vi "Create All Message Queues.vi"(8 "error in (no error)":errorcluster caption="에러 입력(에러 없음)") -> (0 "error out":errorcluster caption="에러 출력", 3 "Message Queues out":T1 caption="메시지 큐 출력")   [LabVIEW 2018, in "Message Queue.lvlib"]
doc: "이 VI는 어플리케이션의 모든 메시지 큐를 생성하고 초기화합니다. 어플리케이션에 하나 이상의 메시지 큐가 필요하면, 위의 \"메시지 큐\" 상수에서 마우스 오른쪽 버튼을 클릭한 후 타입 정의 열기를 선택합니다. 타입 정의에 새 메시지 큐를 추가한 후, 이 VI에서 초기화합니다."
uses:
  Message Queue.lvlib
  All Message Queues.ctl
  Message Cluster.ctl
  Enqueue Message (Single).vi
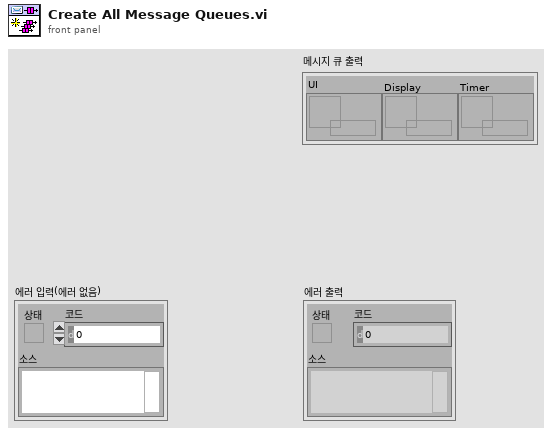
[diagram p1: front panel]
types:
  T1 = typedef "Message Queue.lvlib/All Message Queues.ctl" = cluster{"UI":refnum<queue>, "Display":refnum<queue>, "Timer":refnum<queue>}
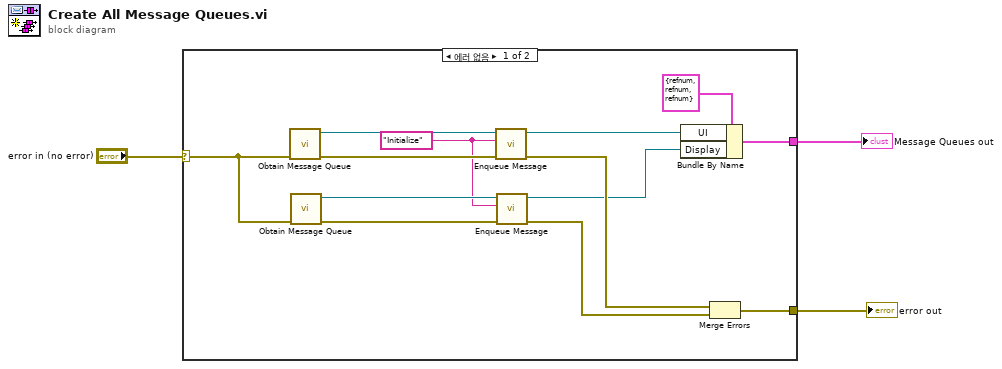
[diagram p0: block diagram]
diagram:
  n1 = case shown="에러 없음" "error in (no error)" {
    selector: "error in (no error)" -> [w5 w17]
    tunnel: [w9 w17] -> w3
    tunnel: [w6 _] -> w2
    frame No Error {
      w4 = "Initialize" ("Message")
      n2 = call "Obtain Message Queue.vi"("error in (no error)"=w5) -> ("error out"=w15:errorcluster, "Message Queue"=w14:refnum<queue>)  [unwired: 9 in]
      n3 = call "Obtain Message Queue.vi"("error in (no error)"=w5) -> ("error out"=w12:errorcluster, "Message Queue"=w13:refnum<queue>)  [unwired: 9 in]
      n4 = call-poly "Enqueue Message.vi"("error in (no error)"=w15, "Message"=w4, "Message Queue"=w14) -> ("error out"=w16:errorcluster, "dup Message Queue"=w11:refnum<queue>)  [unwired: 7 in]
      n5 = call-poly "Enqueue Message.vi"("error in (no error)"=w12, "Message"=w4, "Message Queue"=w13) -> ("error out"=w8:errorcluster, "dup Message Queue"=w10:refnum<queue>)  [unwired: 7 in]
      n6 = Bundle By Name(cluster=T1 {"UI"=refnum, "Display"=refnum, "Timer"=refnum} ("Message Queues"), "UI"=w11, "Display"=w10) -> (w6:T1)
      n7 = Merge Errors(w16, w8) -> (w9:errorcluster)
    }
    frame Error {
    }
  }
  "Message Queues out" <- w2
  "error out" <- w3
